vi "Load_from_Project.vi"(8 "error in (no error)":errorcluster, 9 "index":string, 10 "buildObject":T1, 11 "IB_Destination.lvclass":refnum<class "IB_Destination.lvclass">) -> (0 "error out":errorcluster, 1 "index out":string, 2 "buildObject out":T1, 3 "IB_Destination out":refnum<class "IB_Destination.lvclass">)   [LabVIEW 2020, in "IB_Destination.lvclass"]
uses:
  <vilib>/AppBuilder/IB_Classes/Destination/IB_Destination.lvclass
  <vilib>/AppBuilder/IB_Classes/Destination/IB_Destination.lvclass/IB_Destination.ctl
  <vilib>/AppBuilder/IB_RW_Project/IB_RW_Project_PropBag_Action.ctl
  <resource>/Framework/Providers/API/ItemRef.ctl
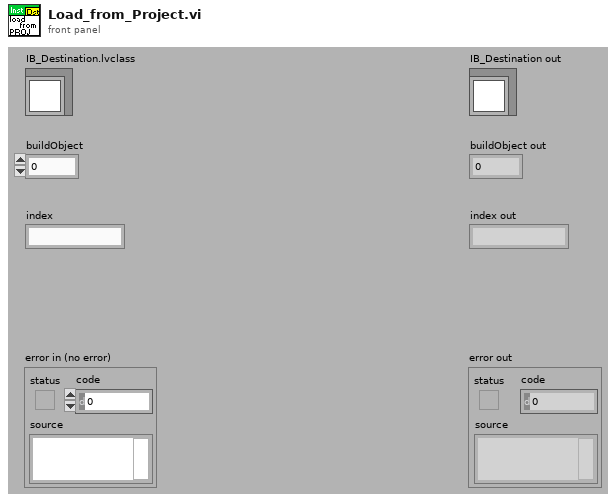
[diagram p1: front panel]
types:
  T1 = typedef "ItemRef.ctl" = u64
  T2 = typedef "IB_RW_Project_PropBag_Action.ctl" = enum16{"read", "write", "clear", "readPrevious", "writePrevious", "clearPrevious"}
  T3 = typedef "IB_RW_Project_Destination_Data.ctl" = cluster{"name":string, "tag":string, "parent":string, "unlock":bool}
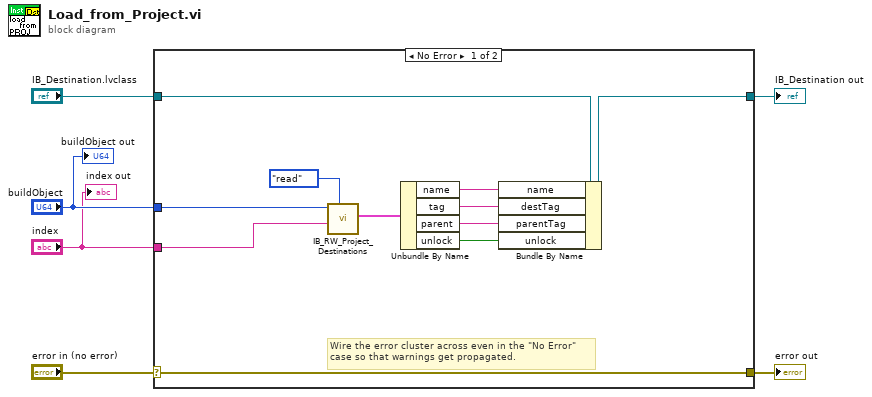
[diagram p0: block diagram]
diagram:
  n1 = case shown="No Error" "error in (no error)" {
    selector: "error in (no error)" -> [w17 w19]
    tunnel: [w17 w19] -> w5
    tunnel: [w7 w18] -> w3
    tunnel: "IB_Destination.lvclass" -> [w8 w18]
    tunnel: "buildObject" -> [w15 _]
    tunnel: "index" -> [w14 _]
    frame No Error {
      # "Wire the error cluster across even in the \"No Error\"\ncase so that warnings get propagated."
      n2 = call <vilib>:"IB_RW_Project_Destinations.vi"("action"=IB_RW_Project_PropBag_Action."read", "index"=w14, "buildObject"=w15) -> ("data"=w13:T3)  [unwired: 5 in, 3 out]
      n3 = Unbundle By Name(w13) -> ("name"=w9:string, "tag"=w10:string, "parent"=w11:string, "unlock"=w12:bool)
      n4 = Bundle By Name(cluster=w8, "name"=w9, "destTag"=w10, "parentTag"=w11, "unlock"=w12) -> (w7:refnum<class "IB_Destination.lvclass">)
    }
    frame Error {
    }
  }
  "error out" <- w5
  "IB_Destination out" <- w3
  "buildObject out" <- "buildObject"
  "index out" <- "index"
